vi "DecodificarGPSRMC.vi"() -> ()   [LabVIEW 2020]
panel:
  out "Fecha":string
  out "Tiempo":string
  out "Longitd":dbl
  out "Latitud":dbl
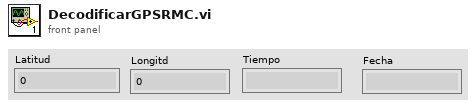
[diagram p1: front panel]
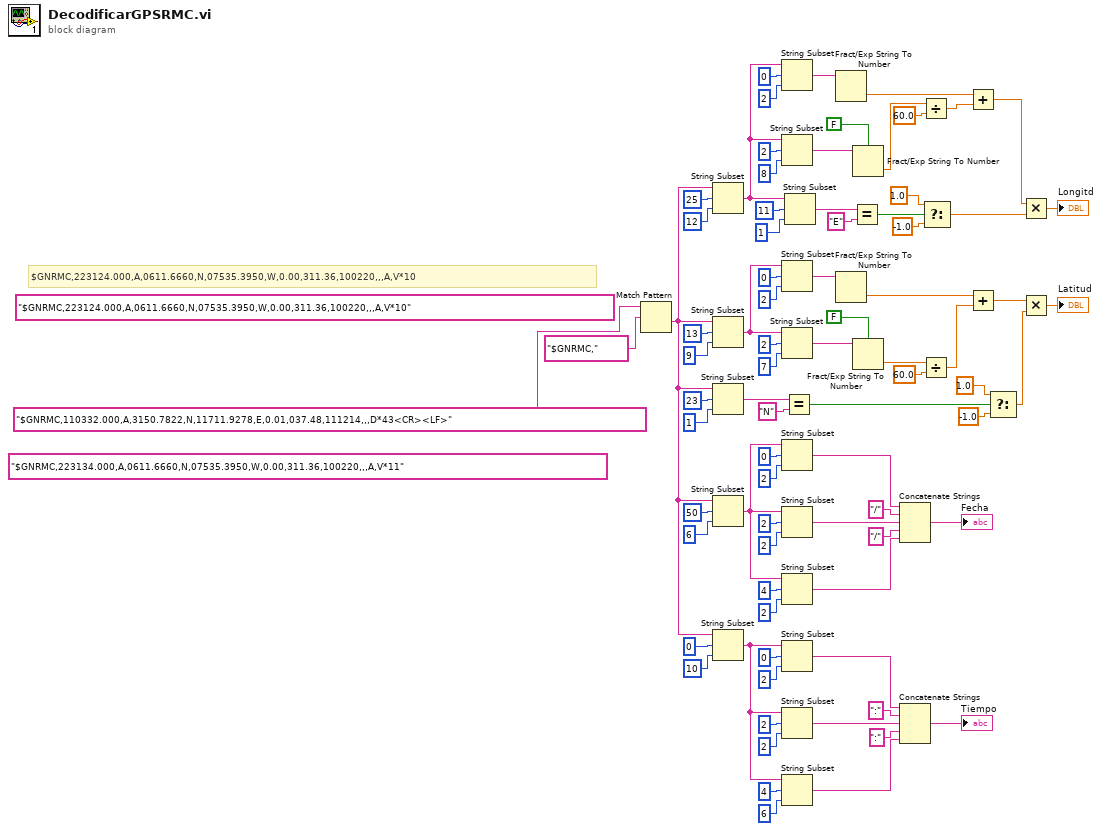
[diagram p0: block diagram]
diagram:
  (unwired) "$GNRMC,223134.000,A,0611.6660,N,07535.3950,W,0.00,311.36,100220,,,A,V*11"
  (unwired) "$GNRMC,223124.000,A,0611.6660,N,07535.3950,W,0.00,311.36,100220,,,A,V*10"
  # "$GNRMC,223124.000,A,0611.6660,N,07535.3950,W,0.00,311.36,100220,,,A,V*10"
  n1 = Match Pattern(string="$GNRMC,110332.000,A,3150.7822,N,11711.9278,E,0.01,037.48,111214,,,D*43<CR><LF>", regular expression="$GNRMC,") -> (after substring=w17:string)  [unwired: 1 in, 3 out]
  n2 = String Subset(string=w17, offset (0)=25, length (rest)=12 ("length (rest)")) -> (substring=w41:string)
  n3 = String Subset(string=w17, offset (0)=13, length (rest)=9 ("length (rest)")) -> (substring=w74:string)
  n4 = String Subset(string=w17, offset (0)=23, length (rest)=1 ("length (rest)")) -> (substring=w64:string)
  n5 = String Subset(string=w17, offset (0)=50, length (rest)=6 ("length (rest)")) -> (substring=w14:string)
  n6 = String Subset(string=w17, offset (0)=0, length (rest)=10 ("length (rest)")) -> (substring=w24:string)
  n7 = String Subset(string=w41, offset (0)=0, length (rest)=2 ("length (rest)")) -> (substring=w54:string)
  n8 = String Subset(string=w41, offset (0)=2, length (rest)=8 ("length (rest)")) -> (substring=w50:string)
  n9 = String Subset(string=w74, offset (0)=0, length (rest)=2 ("length (rest)")) -> (substring=w66:string)
  n10 = String Subset(string=w74, offset (0)=2, length (rest)=7 ("length (rest)")) -> (substring=w71:string)
  n11 = String Subset(string=w14, offset (0)=0, length (rest)=2 ("length (rest)")) -> (substring=w7:string)
  n12 = String Subset(string=w14, offset (0)=2, length (rest)=2 ("length (rest)")) -> (substring=w5:string)
  n13 = String Subset(string=w14, offset (0)=4, length (rest)=2 ("length (rest)")) -> (substring=w3:string)
  n14 = String Subset(string=w24, offset (0)=0, length (rest)=2 ("length (rest)")) -> (substring=w23:string)
  n15 = String Subset(string=w24, offset (0)=2, length (rest)=2 ("length (rest)")) -> (substring=w21:string)
  n16 = String Subset(string=w24, offset (0)=4, length (rest)=6 ("length (rest)")) -> (substring=w19:string)
  n17 = Equal?(x=w64, y="N") -> (x = y?=w62:bool)
  n18 = String Subset(string=w41, offset (0)=11, length (rest)=1 ("length (rest)")) -> (substring=w36:string)
  n19 = Fract/Exp String To Number(string=w54) -> (number=w45:dbl)  [unwired: 3 in, 1 out]
  n20 = Fract/Exp String To Number(string=w66) -> (number=w65:dbl)  [unwired: 3 in, 1 out]
  n21 = Equal?(x=w36, y="E") -> (x = y?=w38:bool)
  n22 = Fract/Exp String To Number(use system decimal point (T)=FALSE, string=w50) -> (number=w52:dbl)  [unwired: 2 in, 1 out]
  n23 = Fract/Exp String To Number(use system decimal point (T)=FALSE, string=w71) -> (number=w69:dbl)  [unwired: 2 in, 1 out]
  n24 = Concatenate Strings(w7, "/" ("string"), w5, "/" ("string"), w3) -> (→"Fecha":string)
  n25 = Concatenate Strings(w23, ":" ("string"), w21, ":" ("string"), w19) -> (→"Tiempo":string)
  n26 = Divide(x=w52, y=60.0) -> (x/y=w44:dbl)
  n27 = Divide(x=w69, y=60.0) -> (x/y=w67:dbl)
  n28 = Select(t=1.0, s=w38, f=-1.0) -> (s? t:f=w35:dbl)
  n29 = Add(x=w45, y=w44) -> (x+y=w34:dbl)
  n30 = Add(x=w65, y=w67) -> (x+y=w58:dbl)
  n31 = Select(t=1.0, s=w62, f=-1.0) -> (s? t:f=w59:dbl)
  n32 = Multiply(x=w34, y=w35) -> (x*y=→"Longitd":dbl)
  n33 = Multiply(x=w58, y=w59) -> (x*y=→"Latitud":dbl)
